vi "Restore Appearance Property.vi"(4 "Control Ref Cluster":T1, 6 "Update?":bool=TRUE, 7 "Polor?":bool, 8 "error in (no error)":errorcluster, 11 "2D Plot.lvclass in":refnum<class "2D Plot.lvclass">) -> (0 "error out":errorcluster, 3 "2D Plot.lvclass out":refnum<class "2D Plot.lvclass">)   [LabVIEW 2017, in "2D Plot.lvclass"]
uses:
  <vilib>/Math Plots/2D Math Plots/2D Plot/2D Plot/2D Plot.lvclass
  <vilib>/Math Plots/2D Math Plots/2D Plot/Action String/2DMathPlot Ctrl Act Cluster.ctl
  <vilib>/Math Plots/2D Math Plots/2D Plot/Action String/2DMathPlot State Class.ctl
  <vilib>/Math Plots/2D Math Plots/2D Plot/2D Plot/2D Plot.lvclass/2D Plot.ctl
  <vilib>/Math Plots/Plot Private Lib/NI_Math Plot Private Lib.lvlib
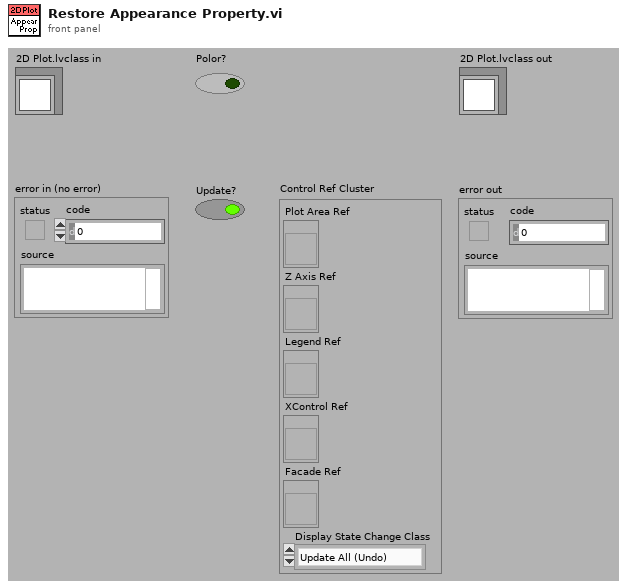
[diagram p1: front panel]
types:
  T1 = typedef "2DMathPlot Ctrl Act Cluster.ctl" = cluster{"Plot Area Ref":refnum<vi>, "Z Axis Ref":refnum<vi>, "Legend Ref":refnum<vi>, "XControl Ref":refnum<vi>, "Facade Ref":refnum<vi>, "Display State Change Class":T2}
  T2 = typedef "2DMathPlot State Class.ctl" = enum16{"Update All (Undo)", "Update General", "Update Appearance", "Update Format", "Update Scale", "Update Marker", "Update Cursor", "None"}
  T3 = cluster{"Left":i16, "Top":i16, "Right":i16, "Bottom":i16}
  T4 = typedef "LVRectTypeDef.ctl" = cluster{"Left":i16, "Top":i16, "Right":i16, "Bottom":i16}
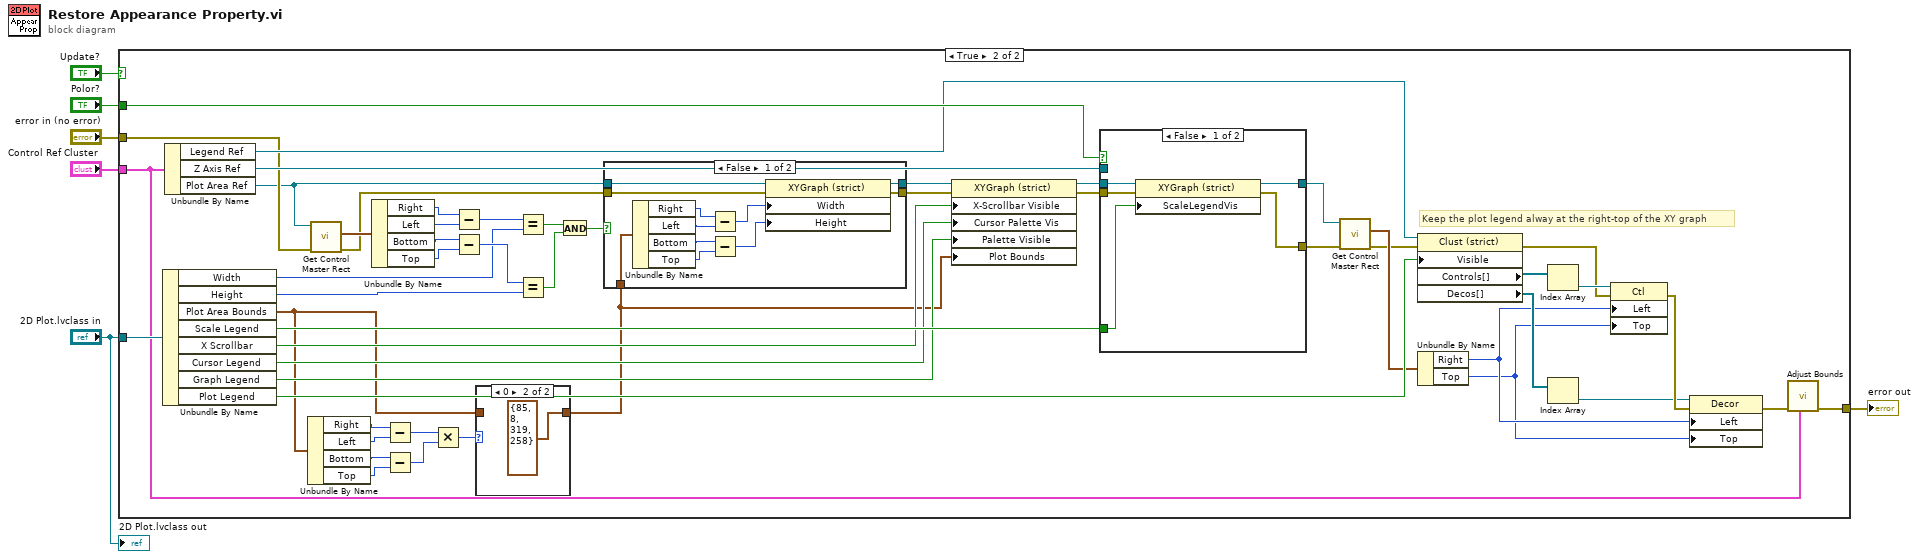
[diagram p0: block diagram]
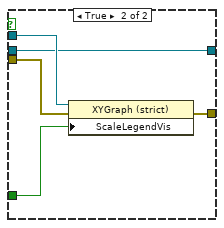
[diagram p5: hidden frame]
diagram:
  n1 = case shown="True" "Update?" {
    tunnel: "2D Plot.lvclass in" -> [_ w49]
    tunnel: [w7 w48] -> w5
    tunnel: "error in (no error)" -> [w7 w25]
    tunnel: "Control Ref Cluster" -> [_ w47]
    tunnel: "Polor?" -> [_ w45]
    frame False {
    }
    frame True {
      # "Keep the plot legend alway at the right-top of the XY graph"
      n2 = Unbundle By Name(w49) -> ("Width"=w17:u32, "Height"=w18:u32, "Plot Area Bounds"=w8:T3, "Scale Legend"=w46:bool, "X Scrollbar"=w42:bool, "Cursor Legend"=w41:bool, "Graph Legend"=w40:bool, "Plot Legend"=w59:bool)
      n3 = Unbundle By Name(w47) -> ("Legend Ref"=w38:refnum<vi>, "Z Axis Ref"=w44:refnum<vi>, "Plot Area Ref"=w24:refnum<vi>)
      n4 = Unbundle By Name(w8) -> ("Right"=w11:i16, "Left"=w12:i16, "Bottom"=w13:i16, "Top"=w14:i16)
      n5 = call <vilib>:"Get Control Master Rect.vi"("error in (no error)"=w25, "reference"=w24) -> ("error out"=w23:errorcluster, "Master Bounds Rect"=w26:T4)  [unwired: 8 out]
      n6 = Unbundle By Name(w26) -> ("Right"=w34:i16, "Left"=w35:i16, "Bottom"=w36:i16, "Top"=w37:i16)
      n7 = Subtract(x=w11, y=w12) -> (x-y=w10:i16)
      n8 = Subtract(x=w13, y=w14) -> (x-y=w9:i16)
      n9 = Multiply(x=w10, y=w9) -> (x*y=w16:i16)
      n10 = Subtract(x=w34, y=w35) -> (x-y=w32:i16)
      n11 = Subtract(x=w36, y=w37) -> (x-y=w33:i16)
      n12 = case shown="0" w16 {
        tunnel: w8 -> [w60 _]
        tunnel: [w60 T3 {"Left"=85, "Top"=8, "Right"=319, "Bottom"=258} ("Plot Area Bounds")] -> w15
        frame Default {
        }
        frame 0 {
        }
      }
      n13 = Equal?(x=w32, y=w17) -> (x = y?=w31:bool)
      n14 = Equal?(x=w33, y=w18) -> (x = y?=w30:bool)
      n15 = And(x=w31, y=w30) -> (x .and. y?=w29:bool)
      n16 = case shown="False" w29 {
        tunnel: w15 -> [w68 _]
        tunnel: w24 -> [w65 w73]
        tunnel: [w64 w73] -> w28
        tunnel: w23 -> [w63 w74]
        tunnel: [w62 w74] -> w27
        frame False {
          n17 = Unbundle By Name(w68) -> ("Right"=w72:i16, "Left"=w71:i16, "Bottom"=w70:i16, "Top"=w69:i16)
          n18 = Subtract(x=w72, y=w71) -> (x-y=w67:i16)
          n19 = Subtract(x=w70, y=w69) -> (x-y=w66:i16)
          n20 = property class="XYGraph (strict)"(reference=w65, error in=w63, "Width"=w67, "Height"=w66) -> (reference out=w64:refnum<vi>, error out=w62:errorcluster)
        }
        frame True {
        }
      }
      n21 = property class="XYGraph (strict)"(reference=w28, error in=w27, "X-Scrollbar Visible"=w42, "Cursor Palette Vis"=w41, "Palette Visible"=w40, "Plot Bounds"=w15) -> (reference out=w43:refnum<vi>, error out=w39:errorcluster)
      n22 = case shown="False" w45 {
        tunnel: w39 -> [w79 w81]
        tunnel: w43 -> [w78 w80]
        tunnel: [w77 w83] -> w21
        tunnel: w46 -> [w76 w82]
        tunnel: w44 -> [_ w84]
        tunnel: [w75 w80] -> w20
        frame False {
          n23 = property class="XYGraph (strict)"(reference=w78, error in=w79, "ScaleLegendVis"=w76) -> (reference out=w75:refnum<vi>, error out=w77:errorcluster)
        }
        frame True {
          n24 = property class="XYGraph (strict)"(reference=w84, error in=w81, "ScaleLegendVis"=w82) -> (error out=w83:errorcluster)  [unwired: 1 out]
        }
      }
      n25 = call <vilib>:"Get Control Master Rect.vi"("error in (no error)"=w21, "reference"=w20) -> ("error out"=w19:errorcluster, "Master Bounds Rect"=w22:T4)  [unwired: 8 out]
      n26 = property class="Clust (strict)"(reference=w38, error in=w19, "Visible"=w59) -> (error out=w56:errorcluster, "Controls[]"=w58:refnum<vi>[], "Decos[]"=w55:refnum<vi>[])  [unwired: 1 out]
      n27 = Unbundle By Name(w22) -> ("Right"=w51:i16, "Top"=w50:i16)
      n28 = Index Array(array=w58) -> (element=w57:refnum<vi>)  [unwired: 1 in]
      n29 = Index Array(array=w55) -> (element=w52:refnum<vi>)  [unwired: 1 in]
      n30 = property class="Ctl"(reference=w57, error in=w56, "Left"=w51, "Top"=w50) -> (error out=w54:errorcluster)  [unwired: 1 out]
      n31 = property class="Decor"(reference=w52, error in=w54, "Left"=w51, "Top"=w50) -> (error out=w53:errorcluster)  [unwired: 1 out]
      n32 = call <vilib>:"Adjust Bounds.vi"("Control Ref Cluster"=w47, "error in (no error)"=w53) -> ("error out"=w48:errorcluster)  [unwired: 9 out]
    }
  }
  "error out" <- w5
  "2D Plot.lvclass out" <- "2D Plot.lvclass in"
